vi "FTW-Scheduler-Destroy.vi"(1 "FTW Job Scheduler":refnum<class "FTW-Scheduler.lvclass">) -> ()   [LabVIEW 2014, in "FTW-Scheduler.lvclass"]
uses:
  FTW-Scheduler.lvclass
panel:
  # "Inputs"
  # "Outputs"
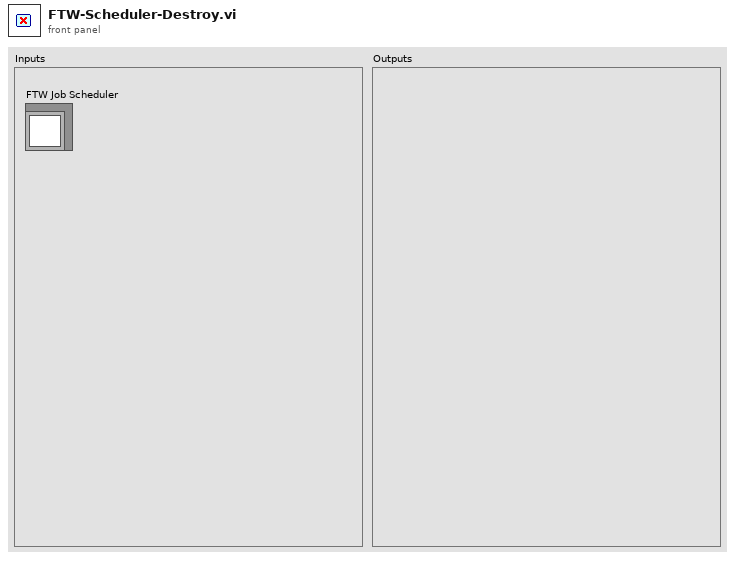
[diagram p1: front panel]
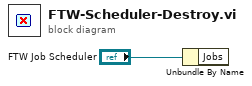
[diagram p0: block diagram]
diagram:
  n1 = Unbundle By Name("FTW Job Scheduler") -> ()  [unwired: 1 out]
